vi "NetComm_SendError.vi"(8 "error in (no error)":errorcluster) -> ()   [LabVIEW 2017]
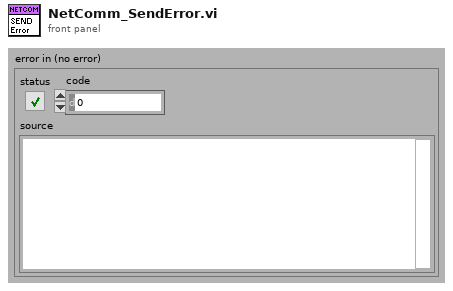
[diagram p1: front panel]
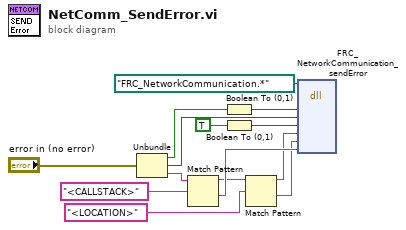
[diagram p0: block diagram]
diagram:
  n1 = Unbundle("error in (no error)") -> ("status"=w12:bool, "code"=w8:i32, "source"=w7:string)
  n2 = Match Pattern(string=w7, regular expression="<CALLSTACK>" ("string")) -> (before substring=w4:string, after substring=w5:string)  [unwired: 1 in, 2 out]
  n3 = Boolean To (0,1)(Boolean=w12) -> (0, 1=w11:i16)
  n4 = Boolean To (0,1)(Boolean=TRUE) -> (0, 1=w10:i16)
  n5 = Match Pattern(string=w4, regular expression="<LOCATION>" ("string")) -> (before substring=w2:string, after substring=w1:string)  [unwired: 1 in, 2 out]
  n6 = dll-call lib="?" fn="FRC_NetworkCommunication_sendError"(path in=path "FRC_NetworkCommunication.*", "isError"=w11, "errorCode"=w8, "isLVCode"=w10, "details"=w2, "location"=w1, "callStack"=w5) -> ()  [unwired: 9 in, 2 out]
